vi "Main.vi"() -> ()   [LabVIEW 2020, in "WebServiceImporter.lvlib" / "Main Panel.lvlib" / "Input WSDL.lvlib"]
uses:
  <vilib>/Platform/WebService/Main Panel/Pages/Input WSDL/Input WSDL.lvlib
  <vilib>/Utility/error.llb/whitespace.ctl
  <vilib>/regexp/Match Regular Expression.xnode
  <vilib>/Platform/WebService/Main Panel/Pages/Input WSDL/Events/Events.lvlib
  <vilib>/Platform/WebService/Main Panel/Pages/Select Methods/Select Methods.lvlib
  <vilib>/Platform/WebService/Main Panel/Pages/Preview/Preview.lvlib
  <vilib>/Platform/WebService/Main Panel/Main Panel.lvlib
  <vilib>/Platform/WebService/ProxyDll Generator/ProxyDll Generator.lvlib
  <vilib>/Platform/WebService/Main Panel/Events/Events.lvlib
  <vilib>/Platform/WebService/Main Panel/Pages/Input Info/Input Info.lvlib
  <vilib>/Platform/WebService/Main Panel/Pages/Authentication/Authentication.lvlib
panel:
  in  "Panel":enum32{"Interface Frame", "Hidden Controls"}(tab)
  in  "Web Service Description Language URL":string
  # "Input the location of a WSDL URL"
  # "Web Service"
  # "Example: http://localhost/DateService.asmx?WSDL"
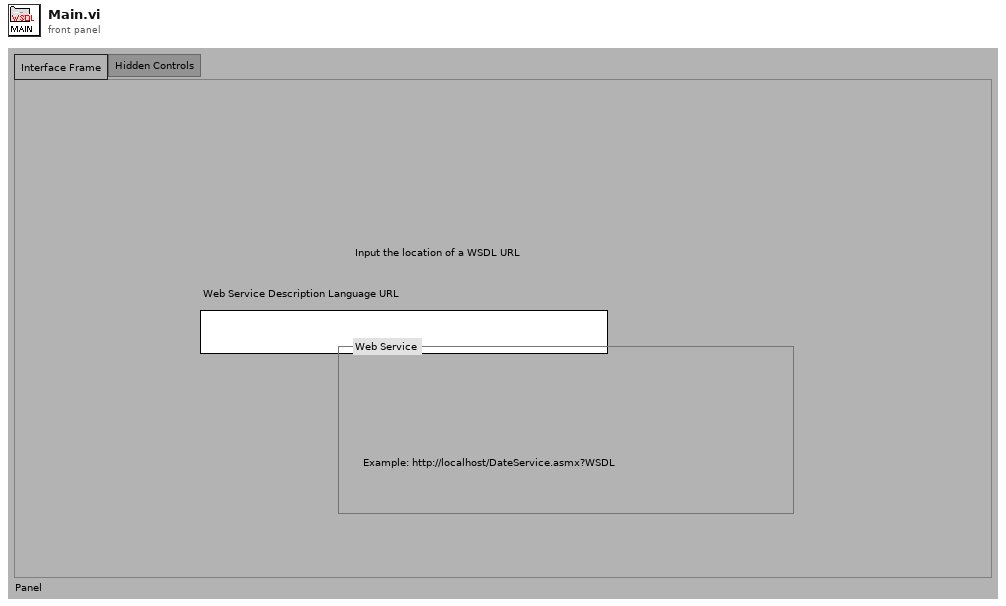
[diagram p1: front panel]
types:
  T1 = enum8{"Enabled", "Disabled", "Disabled and Grayed Out"}
  T2 = typedef "whitespace.ctl" = u16
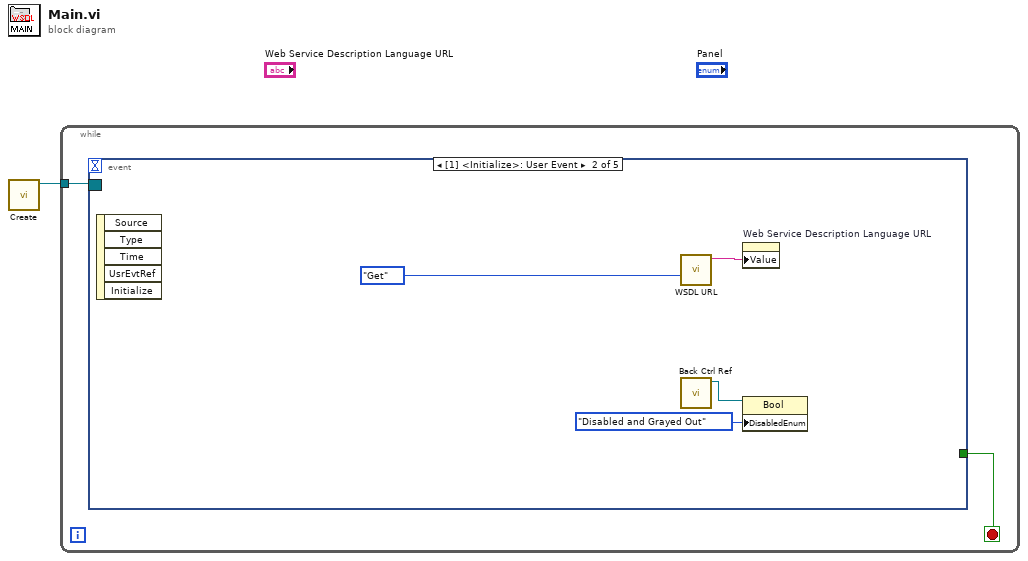
[diagram p0: block diagram]
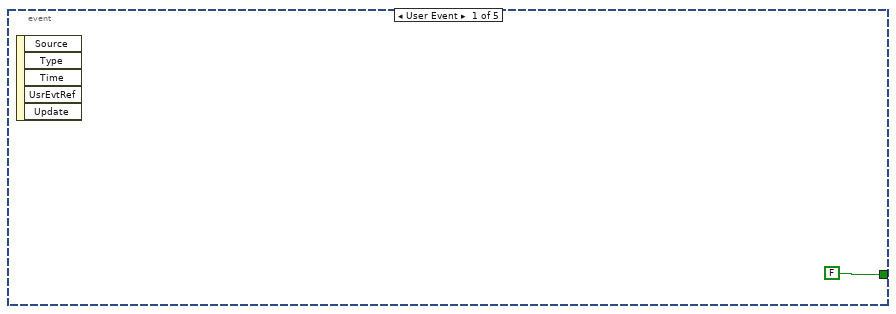
[diagram p2: hidden frame]
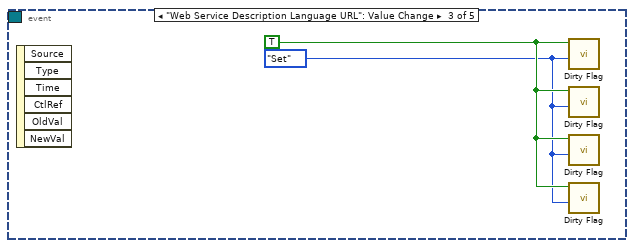
[diagram p3: hidden frame]
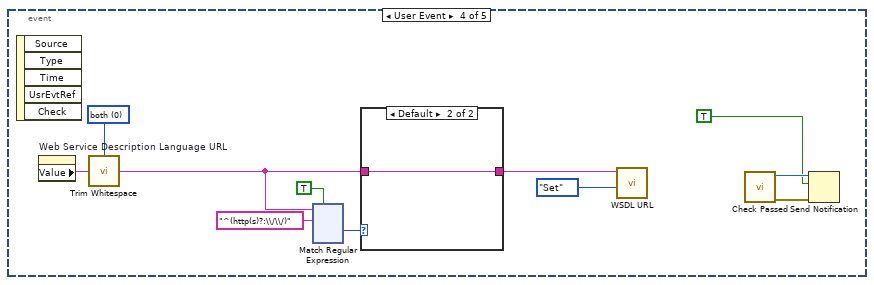
[diagram p4: hidden frame]
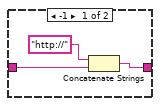
[diagram p5: hidden frame]
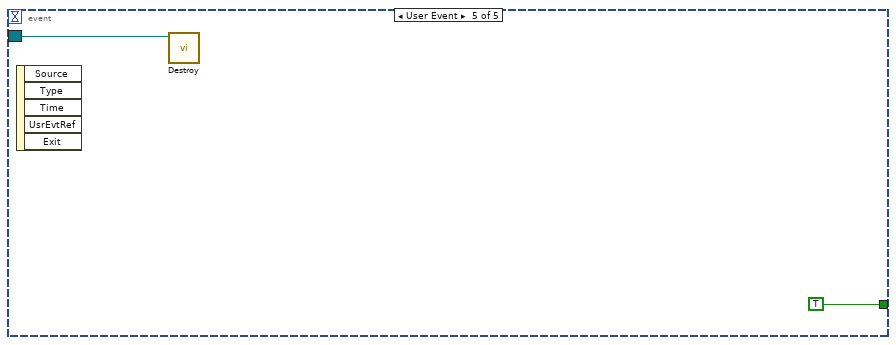
[diagram p6: hidden frame]
diagram:
  n1 = call <vilib>:"Create.vi"() -> ("Event Registration Refnum"=w1:refnum<event-registration>)  [unwired: 10 in, 1 out]
  n2 = while {
    tunnel: w1 -> [w2]
    stop <- w3 stop-if-true
    n3 = event shown="[1] <Initialize>: User Event" {
      selector: w2 -> [_ _ _ _ w138]
      dyn-events: _ -> [_ _ _ _ _]
      timeout: _ -> [_ _ _ _ _]
      tunnel: [FALSE _ _ _ TRUE] -> w3
      event User Event {
        n4 = event-data() -> ()  [unwired: 1 in, 5 out]
      }
      event User Event {
        n5 = event-data() -> ()  [unwired: 1 in, 5 out]
        n6 = call <vilib>:"WSDL URL.vi"("Operation"=enum16{"Get", "Set"}."Get") -> ("WSDL URL (out)"=w7:string)  [unwired: 9 in, 1 out]
        n7 = call <vilib>:"Back Ctrl Ref.vi"() -> ("Ctl Refnum (out)"=w8:refnum<vi>)  [unwired: 10 in, 1 out]
        n8 = property on="Web Service Description Language URL" class="Str"("Value"=w7) -> ()  [unwired: 2 in, 2 out]
        n9 = property class="Bool"(reference=w8, "DisabledEnum"=T1."Disabled and Grayed Out" ("Disabled")) -> ()  [unwired: 1 in, 2 out]
      }
      event "Web Service Description Language URL": Value Change {
        w9 = enum16{"Get", "Set"}."Set" ("Operation")
        w10 = TRUE
        n10 = event-data() -> ()  [unwired: 1 in, 6 out]
        n11 = call <vilib>:"Dirty Flag.vi"("Operation"=w9, "Dirty"=w10) -> ()  [unwired: 8 in, 2 out]
        n12 = call <vilib>:"Dirty Flag.vi"("Operation"=w9, "Dirty"=w10) -> ()  [unwired: 8 in, 2 out]
        n13 = call <vilib>:"Dirty Flag.vi"("Operation"=w9, "Dirty"=w10) -> ()  [unwired: 8 in, 2 out]
        n14 = call <vilib>:"Dirty Flag.vi"("Operation"=w9, "Dirty"=w10) -> ()  [unwired: 8 in, 2 out]
      }
      event User Event {
        w18 = T2 0 items=["both", "start of string", "end of string"] ("location (both)")
        n15 = event-data() -> ()  [unwired: 1 in, 5 out]
        n16 = property on="Web Service Description Language URL" class="Str"() -> ("Value"=w17:string)  [unwired: 2 in, 2 out]
        n17 = call <vilib>:"Trim Whitespace.vi"("string"=w17, "location (both)"=w18) -> ("trimmed string"=w16:string)
        n18 = xnode "Match Regular Expression"("input string"=w16, "regular expression"="^(http(s)?:\\/\\/)" ("search string"), "ignore case? (F)"=TRUE) -> ("offset past match"=w11:i32)  [unwired: 3 in, 4 out]
        n19 = case shown="Default" w11 {
          tunnel: [w134 w136] -> w14
          tunnel: w16 -> [w135 w136]
          frame -1 {
            n20 = Concatenate Strings("http://" ("search string"), w135) -> (w134:string)
          }
          frame Default {
          }
        }
        n21 = call <vilib>:"WSDL URL.vi"("Operation"=enum16{"Get", "Set"}."Set", "WSDL URL"=w14) -> ()  [unwired: 8 in, 2 out]
        n22 = call <vilib>:"Check Passed.vi"() -> ("error out"=w21:errorcluster, "notifier  (out)"=w20:refnum<notifier>)  [unwired: 10 in]
        n23 = Send Notification(notification=TRUE, notifier=w20, error in (no error)=w21) -> ()  [unwired: 2 out]
      }
      event User Event {
        n24 = event-data() -> ()  [unwired: 1 in, 5 out]
        n25 = call <vilib>:"Destroy.vi"("Event Registration Refnum"=w138) -> ()  [unwired: 10 in, 1 out]
      }
    }
  }
